vi "Send Command.vi"(7 "Channel Select":T2, 8 "error in (no error)":errorcluster, 9 "Data":u16, 10 "Power Down Mode":T1, 11 "LINX-DAC8552 in":refnum<class "LINX-DAC8552.lvclass">) -> (0 "error out":errorcluster, 3 "LINX-DAC8552 out":refnum<class "LINX-DAC8552.lvclass">)   [LabVIEW 2020, in "LINX-DAC8552.lvclass"]
doc: "Sends a low-level 3-byte command to the DAC8552."
uses:
  LINX-DAC8552.lvclass
  Channel Select.ctl
  Power Down Mode.ctl
  LINX-DAC8552.lvclass/LINX-DAC8552.ctl
  Read SPI.vi
  Write SPI.vi
  LINX SPI/LINX SPI.lvclass
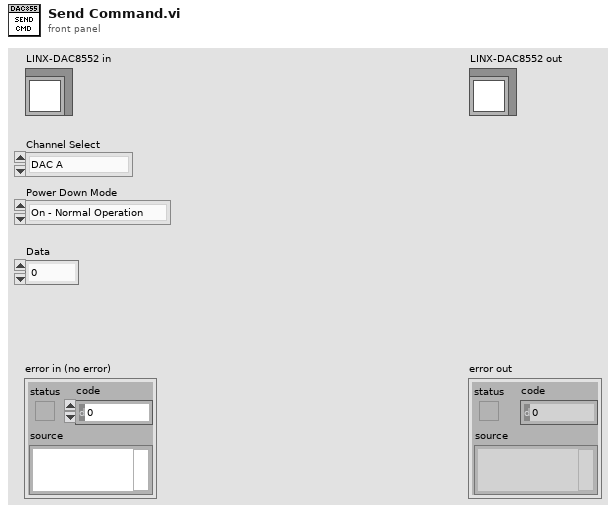
[diagram p1: front panel]
types:
  T1 = typedef "LINX-DAC8552.lvclass/Power Down Mode.ctl" = enum8{"On - Normal Operation", "Off - 1kOhm", "Off - 100kOhm", "Off - High Impedence"}
  T2 = typedef "LINX-DAC8552.lvclass/Channel Select.ctl" = enum8{"DAC A", "DAC B", "Both"}
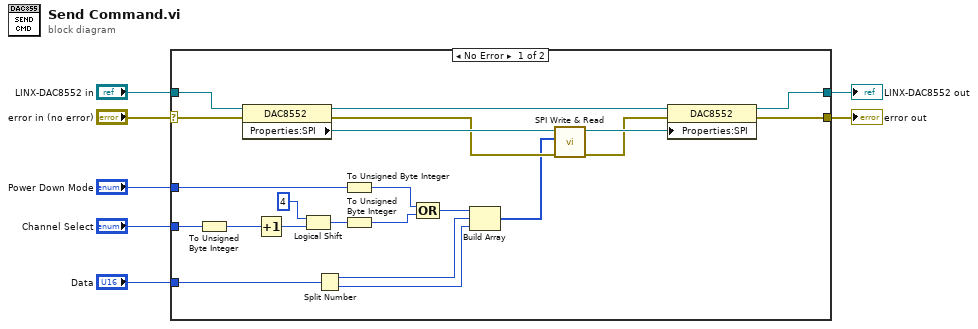
[diagram p0: block diagram]
diagram:
  n1 = case shown="No Error" "error in (no error)" {
    selector: "error in (no error)" -> [w24 w31]
    tunnel: [w13 w31] -> w6
    tunnel: [w27 w30] -> w4
    tunnel: "LINX-DAC8552 in" -> [w29 w30]
    tunnel: "Data" -> [w21 _]
    tunnel: "Channel Select" -> [w9 _]
    tunnel: "Power Down Mode" -> [w14 _]
    frame No Error {
      n2 = To Unsigned Byte Integer(number=w9) -> (unsigned 8bit integer=w8:u8)
      n3 = property class="DAC8552"(reference=w29, error in=w24) -> (reference out=w28:refnum<class "LINX-DAC8552.lvclass">, error out=w23:errorcluster, "Properties:SPI"=w26:refnum<class "LINX SPI.lvclass">)
      n4 = Increment(x=w8) -> (x+1=w16:u8)
      n5 = Logical Shift(y=u8 4 ("hi(x)"), x=w16) -> (x << y=w11:u8)
      n6 = Split Number(x=w21) -> (hi(x)=w19:u8, lo(x)=w20:u8)
      n7 = To Unsigned Byte Integer(number=w14) -> (unsigned 8bit integer=w12:u8)
      n8 = To Unsigned Byte Integer(number=w11) -> (unsigned 8bit integer=w10:u8)
      n9 = Compound Arithmetic op=OR(w12, w10) -> (w17:u8)
      n10 = Build Array(w17, w19, w20) -> (w18:u8[])
      n11 = call "SPI Write & Read.vi"("error in (no error)"=w23, "Data"=w18, "LINX SPI in"=w26) -> ("error out"=w22:errorcluster, "LINX SPI out"=w25:refnum<class "LINX SPI.lvclass">)  [unwired: 6 in, 1 out]
      n12 = property class="DAC8552"(reference=w28, error in=w22, "Properties:SPI"=w25) -> (reference out=w27:refnum<class "LINX-DAC8552.lvclass">, error out=w13:errorcluster)
    }
    frame Error {
    }
  }
  "error out" <- w6
  "LINX-DAC8552 out" <- w4
